vi "_Split Response After Segment Reliability.vi"(0 "Input String":string) -> (1 "Response out":string[](array[string]), 2 "Segment Reliability":i32, 3 "Reliability":i32)   [LabVIEW 2020, in "Rohde&Schwarz CMWXP NR FR1 Measurement.lvlib"]
uses:
  <instrlib>/Rohde&Schwarz CMWXP NR FR1 Measurement/Rohde&Schwarz CMWXP NR FR1 Measurement.lvlib
  <instrlib>/Rohde&Schwarz CMWXP NR FR1 Measurement/Private/rsidr_core.llb/rsidr_core.lvlib
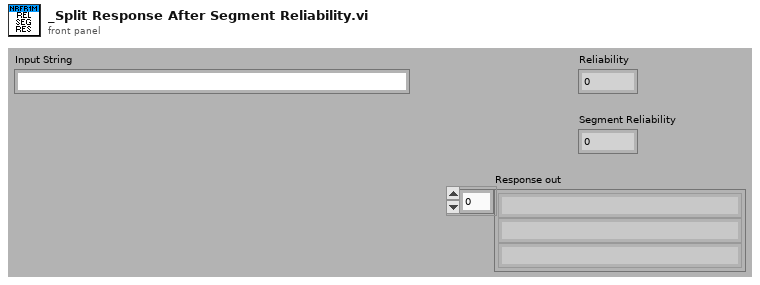
[diagram p1: front panel]
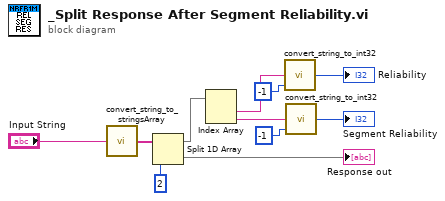
[diagram p0: block diagram]
diagram:
  n1 = call <instrlib>:"convert_string_to_stringsArray.vi"("String in"="Input String") -> ("string array out"=w8:string[])  [unwired: 3 in, 1 out]
  n2 = Split 1D Array(array=w8, index=2) -> (first subarray=w9:string[], second subarray=→"Response out":string[])
  n3 = Index Array(array=w9) -> (element #1=w6:string, element #2=w2:string)  [unwired: 2 in]
  n4 = call <instrlib>:"convert_string_to_int32.vi"("default (0)"=-1 ("default (0 I32)"), "String in"=w6) -> ("int32 value out"=→"Reliability":i32)  [unwired: 3 in]
  n5 = call <instrlib>:"convert_string_to_int32.vi"("default (0)"=-1 ("default (0 I32)"), "String in"=w2) -> ("int32 value out"=→"Segment Reliability":i32)  [unwired: 3 in]
